vi "DOConfigureClock.vi"(0 "object in":refnum<class "AD2_DO_SDK.lvclass">, 1 "DO Trigger":T2, 2 "ClockSettings":T1(array[cluster]), 5 "error in (no error)":errorcluster) -> (14 "object out":refnum<class "AD2_DO_SDK.lvclass">, 19 "error out":errorcluster)   [LabVIEW 2024, in "AD2_DO_SDK.lvclass"]
uses:
  AD2_DO_SDK.lvclass
  DOTrigger.ctl
  AD2_WFG_SDK_class/AD2TriggerSources.ctl
  AD2_DO_SDK.lvclass/AD2_DO_SDK.ctl
  AD2_SDK_class/AD2_SDK.lvclass
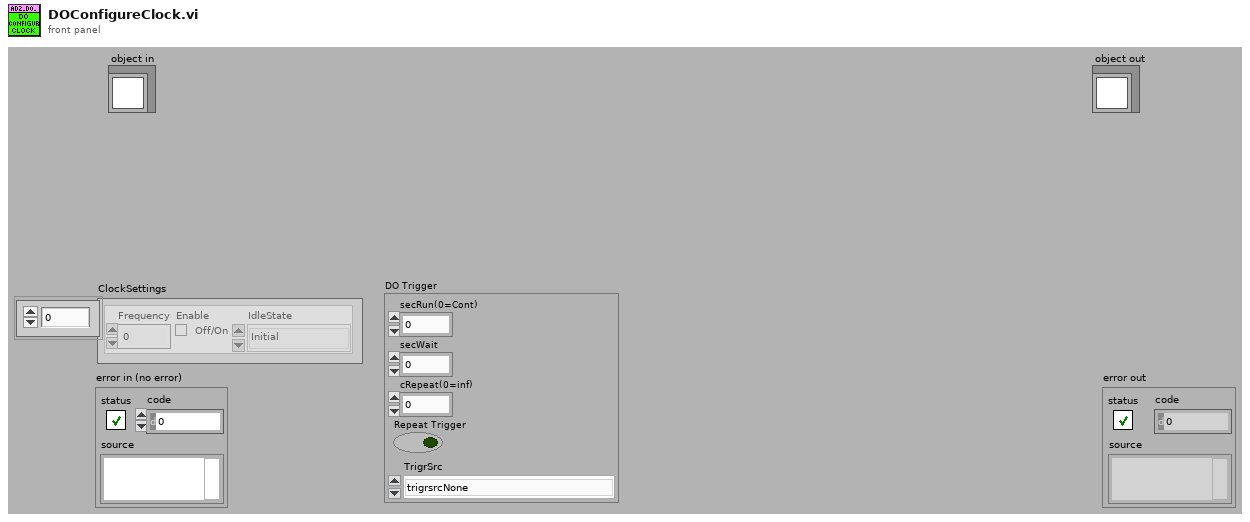
[diagram p1: front panel]
types:
  T1 = cluster{"Frequency":dbl, "Enable":bool, "IdleState":enum16{"Initial", "Low", "High", "Z"}}[]
  T2 = typedef "AD2_DO_SDK.lvclass/DOTrigger.ctl" = cluster{"secRun(0=Cont)":dbl, "secWait":dbl, "cRepeat(0=inf)":i32, "Repeat Trigger":bool, "TrigrSrc":T3}
  T3 = typedef "AD2_SDK.lvclass/AD2TriggerSources.ctl" = enum8{"trigrsrcNone", "trigsrcPC", "trigsrcDetectorAnalogIn", "trigsrcDetectorDigitalIn", "trigsrcAnalogIn", "trigsrcDigitalIn", "trigsrcDigitalOut", "trigsrcAnalogOut1", "trigsrcAnalogOut2", "trigsrcAnalogOut3", "trigsrcAnalogOut4", "trigsrcExternal1", "trigsrcExternal2", "trigsrcExternal3", "trigsrcExternal4", ""}
  T4 = cluster{"NoHighBits":u32, "NoLowBits":u32, "NoInitialBits":u32, "Start High":bool}
  T5 = typedef "AD2_DO_SDK.lvclass/DOSingleCh.ctl" = cluster{"Ch Index":i32, "Enable":bool, "Clock DIvider":u32, "Type":i32, "DigitalOutOutput":u16, "IdleState":u16, "CounterData":cluster{"NoHighBits":u32, "NoLowBits":u32, "NoInitialBits":u32, "Start High":bool}, "Custom Data":cluster{"countOfBits":u32, "rgBits":u8[]}}
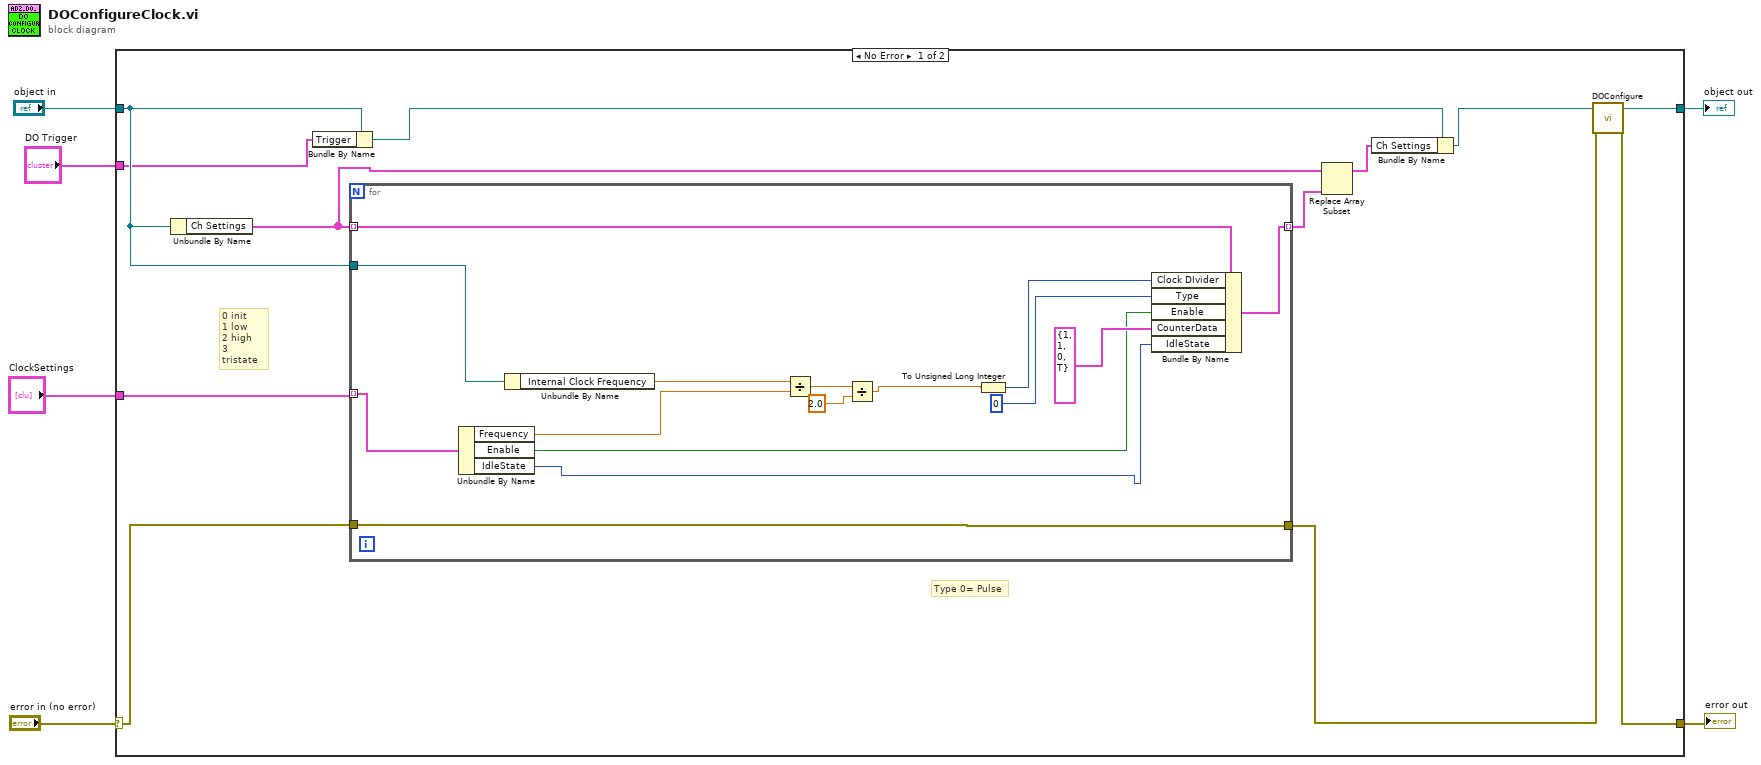
[diagram p0: block diagram]
diagram:
  n1 = case shown="No Error" "error in (no error)" {
    selector: "error in (no error)" -> [w14 w35]
    tunnel: [w18 w35] -> w5
    tunnel: [w17 w34] -> w3
    tunnel: "object in" -> [w12 w34]
    tunnel: "DO Trigger" -> [w11 _]
    tunnel: "ClockSettings" -> [w10 _]
    frame No Error {
      # "0 init\n1 low\n2 high\n3 tristate"
      # "Type 0= Pulse"
      n2 = Unbundle By Name(w12) -> ("Ch Settings"=w9:T5[])
      n3 = Bundle By Name(cluster=w12, "Trigger"=w11) -> (w13:refnum<class "AD2_DO_SDK.lvclass">)
      n4 = for {
        tunnel: w9 -> [w27] mode=indexing
        tunnel: [w33] -> w8 mode=indexing
        tunnel: w14 -> [w23]
        tunnel: [w23] -> w15
        tunnel: w12 -> [w32]
        tunnel: w10 -> [w22] mode=indexing
        n5 = Unbundle By Name(w22) -> ("Frequency"=w21:dbl, "Enable"=w20:bool, "IdleState"=w19:enum16{"Initial", "Low", "High", "Z"})
        n6 = Unbundle By Name(w32) -> ("Internal Clock Frequency"=w31:dbl)
        n7 = Divide(x=w31, y=w21) -> (x/y=w25:dbl)
        n8 = Divide(x=w25, y=2.0) -> (x/y=w24:dbl)
        n9 = To Unsigned Long Integer(number=w24) -> (unsigned 32bit integer=w30:u32)
        n10 = Bundle By Name(cluster=w27, "Clock DIvider"=w30, "Type"=0, "Enable"=w20, "CounterData"=T4 {"NoHighBits"=1, "NoLowBits"=1, "NoInitialBits"=0, "Start High"=TRUE}, "IdleState"=w19) -> (w33:T5)
      }
      n11 = Replace Array Subset(array=w9, new element=w8) -> (w7:T5[])  [unwired: 1 in]
      n12 = Bundle By Name(cluster=w13, "Ch Settings"=w7) -> (w16:refnum<class "AD2_DO_SDK.lvclass">)
      n13 = call-dynamic "DOConfigure.vi"("object in"=w16, "error in (no error)"=w15) -> ("object out"=w17:refnum<class "AD2_DO_SDK.lvclass">, "error out"=w18:errorcluster)  [unwired: 16 in]
    }
    frame Error {
    }
  }
  "error out" <- w5
  "object out" <- w3
